vi "from string 1.0.vi"(8 "error in (no error)":errorcluster, 10 "data":string, 11 "OnTheFlyReport Config in":refnum<class "OnTheFlyReport Config.lvclass">) -> (0 "error out":errorcluster, 3 "OnTheFlyReport Config out":refnum<class "OnTheFlyReport Config.lvclass">)   [LabVIEW 2015, in "OnTheFlyReport Config.lvclass"]
uses:
  OnTheFlyReport Config.lvclass
  OnTheFlyReport Config.lvclass/OnTheFlyReport Config.ctl
  Report Formatters/Base Class/Config/Formatter Config.lvclass
  <vilib>/NI/Configuration Framework/serializable configuration/NISE_CEF_serializable configuration.lvclass
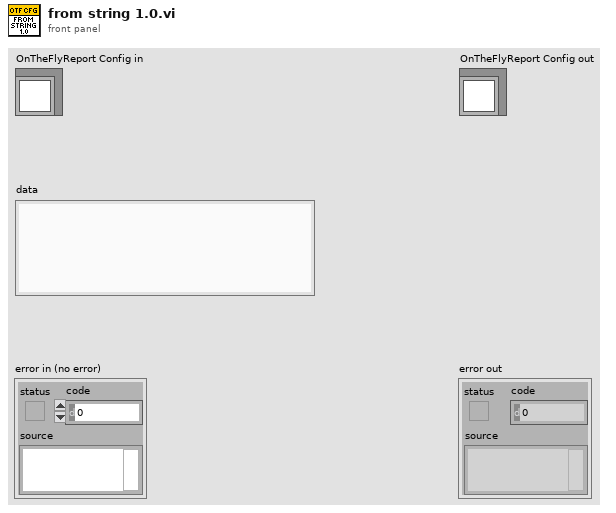
[diagram p1: front panel]
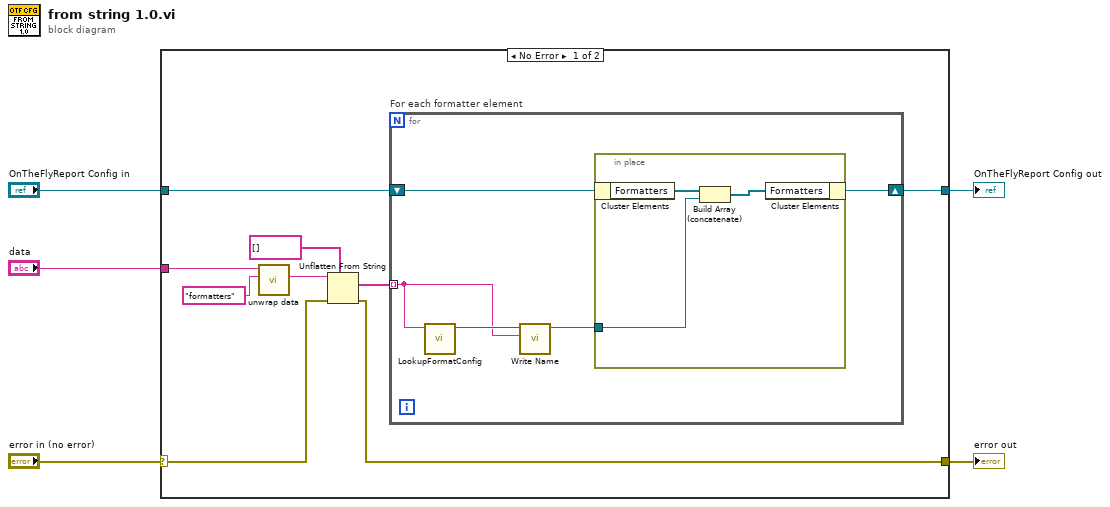
[diagram p0: block diagram]
diagram:
  n1 = case shown="No Error" "error in (no error)" {
    selector: "error in (no error)" -> [w8 w24]
    tunnel: [w7 w24] -> w4
    tunnel: [w13 w23] -> w3
    tunnel: "OnTheFlyReport Config in" -> [w14 w23]
    tunnel: "data" -> [w12 _]
    frame No Error {
      n2 = call <vilib>:"unwrap data.vi"("identifier"="formatters", "data to unwrap"=w12) -> ("unwrapped data"=w9:string)  [unwired: 8 in, 1 out]
      n3 = Unflatten From String(type=string[] [], binary string=w9, error in (no error)=w8) -> (value=w6:string[], error out=w7:errorcluster)  [unwired: 2 in, 1 out]
      n4 = for "For each formatter element" {
        shift-right: [w18] -> w13
        shift-left: w14 -> [w19]
        tunnel: w6 -> [w15] mode=indexing
        n5 = call "LookupFormatConfig.vi"("format string"=w15) -> ("Formatter Config out"=w17:refnum<class "Formatter Config.lvclass">)  [unwired: 10 in]
        n6 = call-dynamic "Write Name.vi"("Name"=w15, "Formatter Config in"=w17) -> ("Formatter Config out"=w16:refnum<class "Formatter Config.lvclass">)  [unwired: 8 in, 1 out]
        n7 = in-place {
          in-place-border: w16 -> [w20]
          n8 = in-place-cluster #1(w19) -> ("Formatters"=w22:refnum<class "Formatter Config.lvclass">[])
          n9 = Build Array (concatenate)(w22, w20) -> (w21:refnum<class "Formatter Config.lvclass">[])
          n10 = in-place-cluster #1("Formatters"=w21) -> (w18:refnum<class "OnTheFlyReport Config.lvclass">)
        }
      }
    }
    frame Error {
    }
  }
  "error out" <- w4
  "OnTheFlyReport Config out" <- w3
